vi "Alpha 5.0.1.vi"() -> ()   [LabVIEW 2011]
panel:
  out "Path to Image":path
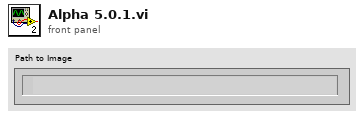
[diagram p1: front panel]
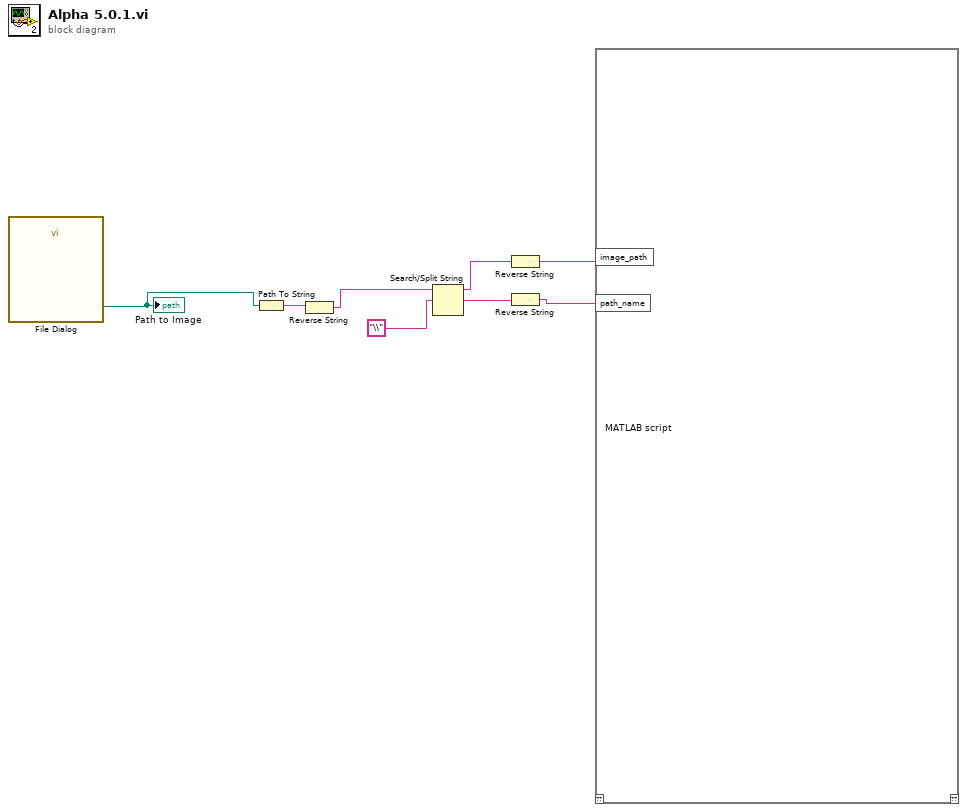
[diagram p0: block diagram]
diagram:
  n1 = call "File Dialog"() -> ("selected path"=w8:path)  [unwired: 12 in, 3 out]
  "Path to Image" <- w8
  n2 = Path To String(path=w8) -> (string=w7:string)
  n3 = Reverse String(1:w7) -> (0:w6:string)
  n4 = Search/Split String(string=w6, search string/char (-)="\\") -> (substring before match=w4:string, match + rest of string=w3:string)  [unwired: 1 in, 1 out]
  n5 = Reverse String(1:w4) -> (0:w2:string)
  n6 = Reverse String(1:w3) -> (0:w1:string)
  n7 = script code="MATLAB script"("image_path"=w2, "path_name"=w1) -> ()  [unwired: 1 in, 1 out]
